vi "m1m3_logEvent_DetailedState.vi"(8 "error in (no error)":errorcluster, 11 "logevent_DetailedState_Ctl":T1) -> (0 "error out":errorcluster, 2 "function return":i32, 3 "logevent_DetailedState_Ctl out":T1)   [LabVIEW 2016, in "SALLV_m1m3.lvlib"]
doc: "int m1m3_shm_logEvent_DetailedStateLV(m1m3_logevent_DetailedStateLV *logevent_DetailedState_Ctl );"
uses:
  SALLV_m1m3.lvlib
  DataTypes/logevent_DetailedState.ctl
  SALLV_m1m3.so
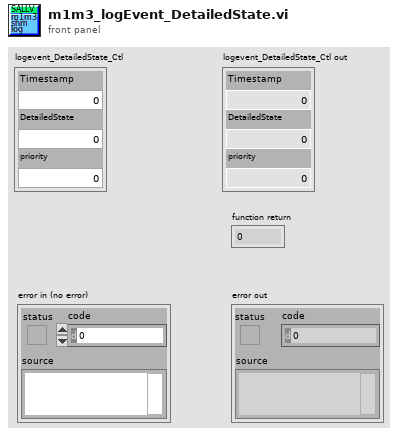
[diagram p1: front panel]
types:
  T1 = typedef "SALLV_m1m3.lvlib/logevent_DetailedState.ctl" = cluster{"Timestamp":dbl, "DetailedState":i32, "priority":i32}
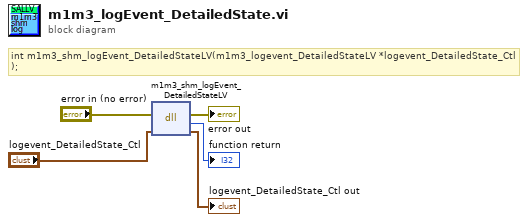
[diagram p0: block diagram]
diagram:
  # "int m1m3_shm_logEvent_DetailedStateLV(m1m3_logevent_DetailedStateLV *logevent_DetailedState_Ctl );"
  n1 = dll-call lib="opt/CODE/SALLV_m1m3/SALLV_m1m3.*" fn="m1m3_shm_logEvent_DetailedStateLV"(error in="error in (no error)", "logevent_DetailedState_Ctl"="logevent_DetailedState_Ctl") -> (error out=→"error out":errorcluster, →"function return":i32, "logevent_DetailedState_Ctl"=→"logevent_DetailedState_Ctl out":T1)  [unwired: 2 in, 1 out]
